vi "pascal triangle.vi"() -> ()   [LabVIEW 2017]
panel:
  in  "Numeric":dbl
  out "String":string
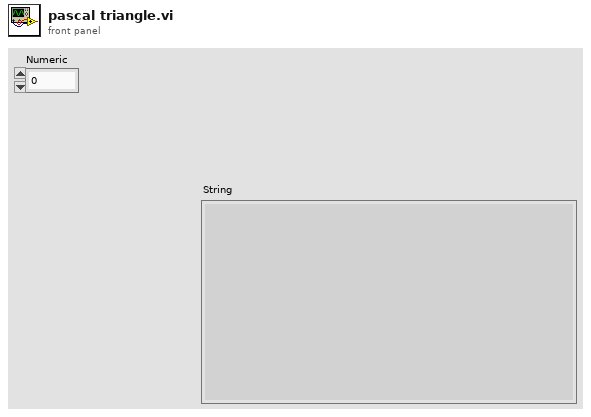
[diagram p1: front panel]
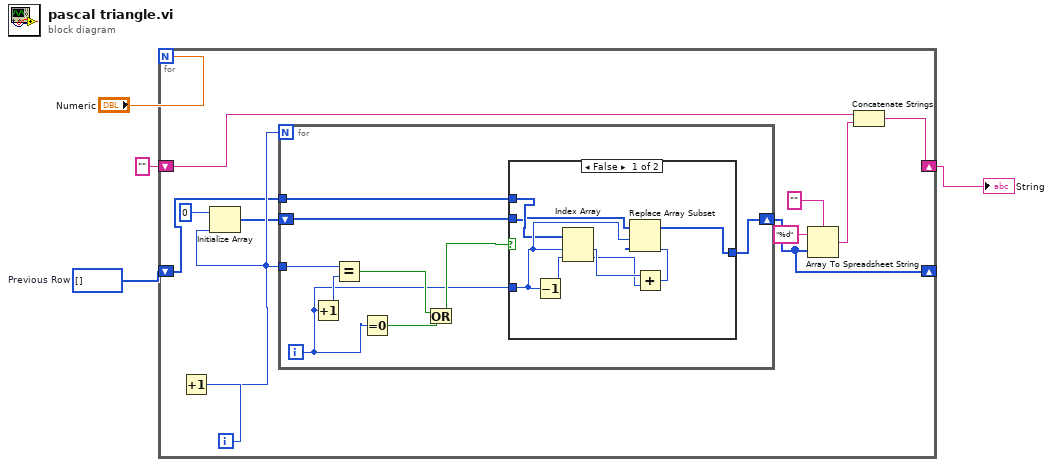
[diagram p0: block diagram]
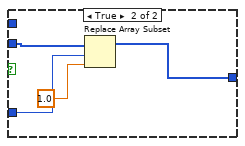
[diagram p2: hidden frame]
diagram:
  w1 = i32[] []  # Previous Row
  n1 = for {
    N: "Numeric" -> [_]
    shift-right: [w9] -> w3
    shift-left: "" -> [w10]
    shift-right: [w5] -> _
    shift-left: w1 -> [w8]
    i -> [w15]
    n2 = Increment(x=w15) -> (x+1=w14:i32)
    n3 = Initialize Array(0, w14) -> (w12:i32[])
    n4 = for {
      N: w14 -> [_]
      tunnel: w14 -> [w22]
      shift-right: [w19] -> w5
      shift-left: w12 -> [w18]
      tunnel: w8 -> [w16]
      i -> [w17]
      n5 = Increment(x=w17) -> (x+1=w23:i32)
      n6 = Equal?(x=w22, y=w23) -> (x = y?=w21:bool)
      n7 = Equal To 0?(x=w17) -> (x = 0?=w24:bool)
      n8 = Or(x=w21, y=w24) -> (x .or. y?=w20:bool)
      n9 = case shown="False" w20 {
        tunnel: [w27 w35] -> w19
        tunnel: w18 -> [w25 w34]
        tunnel: w17 -> [w28 w33]
        tunnel: w16 -> [w26 _]
        frame False {
          n10 = Decrement(x=w28) -> (x-1=w32:i32)
          n11 = Index Array(array=w26, index #1=w28, index #2=w32) -> (element #1=w31:i32, element #2=w30:i32)
          n12 = Add(x=w31, y=w30) -> (x+y=w29:i32)
          n13 = Replace Array Subset(array=w25, new element=w29, index=w28) -> (w27:i32[])
        }
        frame True {
          n14 = Replace Array Subset(array=w34, new element=1.0 ("new element/subarray"), index=w33) -> (w35:i32[])
        }
      }
    }
    n15 = Array To Spreadsheet String(delimiter (Tab)="", array=w5, 3:"%d" ("format string")) -> (spreadsheet string=w11:string)
    n16 = Concatenate Strings(w10, w11) -> (w9:string)
  }
  "String" <- w3
